vi "Write.vi"(10 "Path":path, 11 "Path in":refnum<class "Path.lvclass">) -> (3 "Path out":refnum<class "Path.lvclass">)   [LabVIEW 2020, in "Data.lvlib" / "Path.lvclass"]
doc: "Write string."
uses:
  Path.lvclass
  Path.lvclass/Path.ctl
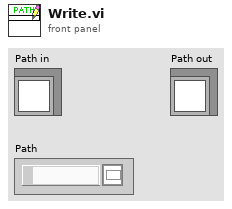
[diagram p1: front panel]
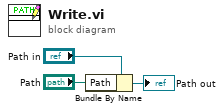
[diagram p0: block diagram]
diagram:
  n1 = Bundle By Name(cluster="Path in", "Path"="Path") -> (→"Path out":refnum<class "Path.lvclass">)
